vi "MathOptim-Logistic Full Parameter Vector.vi"(0 "Y":dbl[](array[numeric]), 5 "X":dbl[](array[numeric]), 7 "a":dbl[](array[numeric])) -> (8 "Parameters":dbl[](array[numeric]))   [LabVIEW 2015]
doc: "This template is the starting point for creating a model function to be passed to the Nonlinear Curve Fit.vi."
uses:
  <vilib>/Analysis/7linalg.llb/Solve Linear Equations (single right hand).vi
  <vilib>/Analysis/baseanly.llb/Solve Linear Equations By Cholesky.vi
  <vilib>/Analysis/baseanly.llb/Real Matrix to Compact Array.vi
  <vilib>/Analysis/baseanly.llb/Real Compact Tri-Matrix Linear Eqs.vi
  <vilib>/Analysis/7linalg.llb/Solve Linear Eqs (General).vi
  <vilib>/Analysis/7linalg.llb/Solve Linear Eqs (Gen, single right hand).vi
  <vilib>/Analysis/NI_AALPro.lvlib
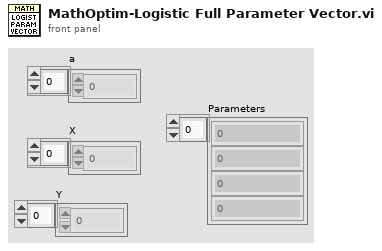
[diagram p1: front panel]
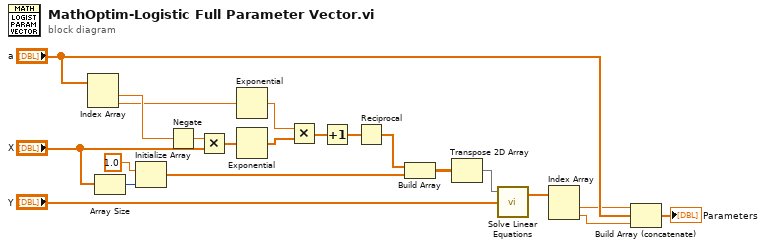
[diagram p0: block diagram]
diagram:
  n1 = Index Array(array="a") -> (element #1=w14:dbl, element #2=w12:dbl)  [unwired: 2 in]
  n2 = Array Size(array="X") -> (size(s)=w21:i32)
  n3 = Initialize Array(1.0, w21) -> (w19:dbl[])
  n4 = Negate(x=w14) -> (-x=w1:dbl)
  n5 = Multiply(x=w1, y="X") -> (x*y=w13:dbl[])
  n6 = Exponential(1:w12) -> (0:w11:dbl)
  n7 = Exponential(1:w13) -> (0:w10:dbl[])
  n8 = Multiply(x=w11, y=w10) -> (x*y=w9:dbl[])
  n9 = Increment(x=w9) -> (x+1=w8:dbl[])
  n10 = Reciprocal(x=w8) -> (1/x=w7:dbl[])
  n11 = Build Array(w7, w19) -> (w18:dbl[][])
  n12 = Transpose 2D Array(2D array=w18) -> (transposed array=w16:dbl[][])
  n13 = call-poly <vilib>:"Solve Linear Equations.vi"("Known Vector"="Y", "Input Matrix"=w16) -> ("Solution Vector"=w17:dbl[])  [unwired: 1 in, 1 out]
  n14 = Index Array(array=w17) -> (element #1=w4:dbl, element #2=w3:dbl)  [unwired: 2 in]
  n15 = Build Array (concatenate)(w4, "a", w3) -> (→"Parameters":dbl[])
